vi "DAQ_pp3c_AllInit.vi"(8 "error in (no error)":errorcluster, 11 "Daq config in":T1={"Sound AO"="Dev6/ao0", "Shock intesity AO"="Dev6/ao1", "Code_LED DO"="Dev6/port1:2", "Switch DI"="Dev6/port0/line0", "Webcam"="cam9", "Sound AO task"="", "Sound card task"=0, "Shock intensity AO task"="", "Code_LED DO task"="", "Switch DI task"="", "AO <=> Sound card"=FALSE, "Sound card"=0, "sample rate"=100000.0, "Variable shock"=TRUE, "Webcam on"=FALSE, "Waveform memo"={"t0"=timestamp(0 s since 1904-01-01), "dt"=1.0, "Y"=[]}, "Tone trigger"="PFI1", "Master-9 DO"="PFI1", "Master-9 DO task"="Dev6/port0/line5:7", "Master-9 on"=TRUE} {"sample rate" min=8000.0; "Sound card task" format="%.0x"}) -> (0 "error out":errorcluster={"status"=FALSE, "code"=0, "source"="\n"}, 3 "Daq config out":T1={"Sound AO"="Dev6/ao0", "Shock intesity AO"="Dev6/ao1", "Code_LED DO"="Dev6/port1:2", "Switch DI"="Dev6/port0/line0", "Webcam"="cam9", "Sound AO task"="", "Sound card task"=0, "Shock intensity AO task"="", "Code_LED DO task"="", "Switch DI task"="", "AO <=> Sound card"=FALSE, "Sound card"=0, "sample rate"=100000.0, "Variable shock"=TRUE, "Webcam on"=FALSE, "Waveform memo"={"t0"=timestamp(0 s since 1904-01-01), "dt"=1.0, "Y"=[]}, "Tone trigger"="PFI1", "Master-9 DO"="PFI1", "Master-9 DO task"="Dev6/port0/line5:7", "Master-9 on"=TRUE} {"sample rate" min=8000.0; "Sound card task" format="%.0x"})   [LabVIEW 2013]
uses:
  CTL_pp3c_DaqStatus.ctl
  <vilib>/userdefined/High Color/IMAQdx.ctl
  <vilib>/sound2/lvsound2.llb/Sound Output Task ID.ctl
  <vilib>/sound2/lvsound2.llb/Sampling Mode.ctl
  <vilib>/sound2/lvsound2.llb/Sound Data Format.ctl
  <vilib>/DAQmx/write.llb/DAQmx Write (Digital U16 1Chan 1Samp).vi
  <vilib>/DAQmx/write.llb/DAQmx Write (Digital U32 1Chan 1Samp).vi
  <vilib>/DAQmx/create/channels.llb/DAQmx Create Channel (DO-Digital Output).vi
  <vilib>/DAQmx/create/channels.llb/DAQmx Create Channel (DI-Digital Input).vi
  <vilib>/DAQmx/create/channels.llb/DAQmx Create Channel (AO-Voltage-Basic).vi
  <vilib>/DAQmx/configure/timing.llb/DAQmx Timing (Sample Clock).vi
  <vilib>/DAQmx/miscellaneous.llb/DAQmx Fill In Error Info.vi
  <resource>/objmgr/daqmx.rc
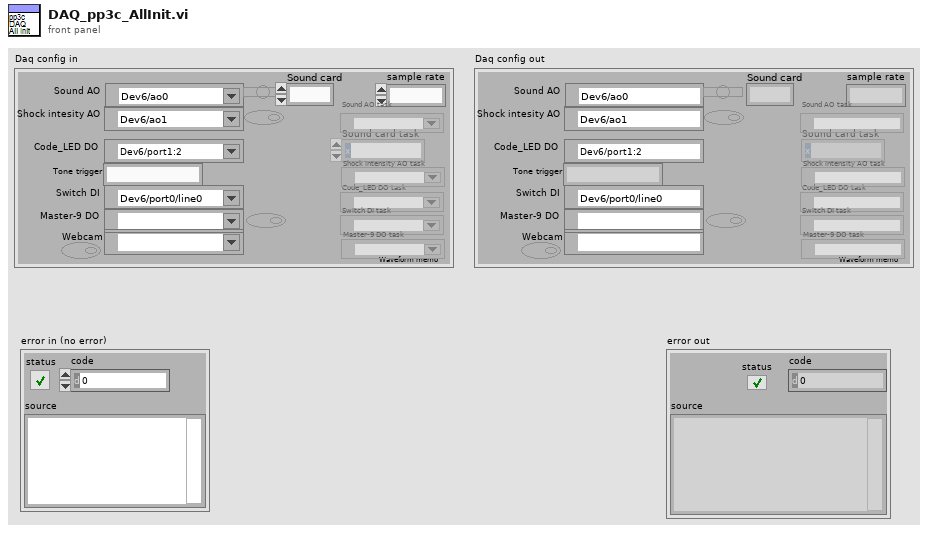
[diagram p1: front panel]
types:
  T1 = typedef "CTL_pp3c_DaqStatus.ctl" = cluster{"Sound AO":tag, "Shock intesity AO":tag, "Code_LED DO":tag, "Switch DI":tag, "Webcam":T2, "Sound AO task":refnum<k21>, "Sound card task":T3, "Shock intensity AO task":refnum<k21>, "Code_LED DO task":refnum<k21>, "Switch DI task":refnum<k21>, "AO <=> Sound card":bool, "Sound card":u32, "sample rate":dbl, "Variable shock":bool, "Webcam on":bool, "Waveform memo":waveform(dbl), "Tone trigger":string, "Master-9 DO":tag, "Master-9 DO task":refnum<k21>, "Master-9 on":bool}
  T2 = typedef "IMAQdx.ctl" = refnum<k21>
  T3 = typedef "Sound Output Task ID.ctl" = u32
  T4 = typedef "Sound Data Format.ctl" = cluster{"sample rate (S/s)":dbl, "number of channels":i32, "bits per sample":i32}
  T5 = typedef "Sampling Mode.ctl" = i32
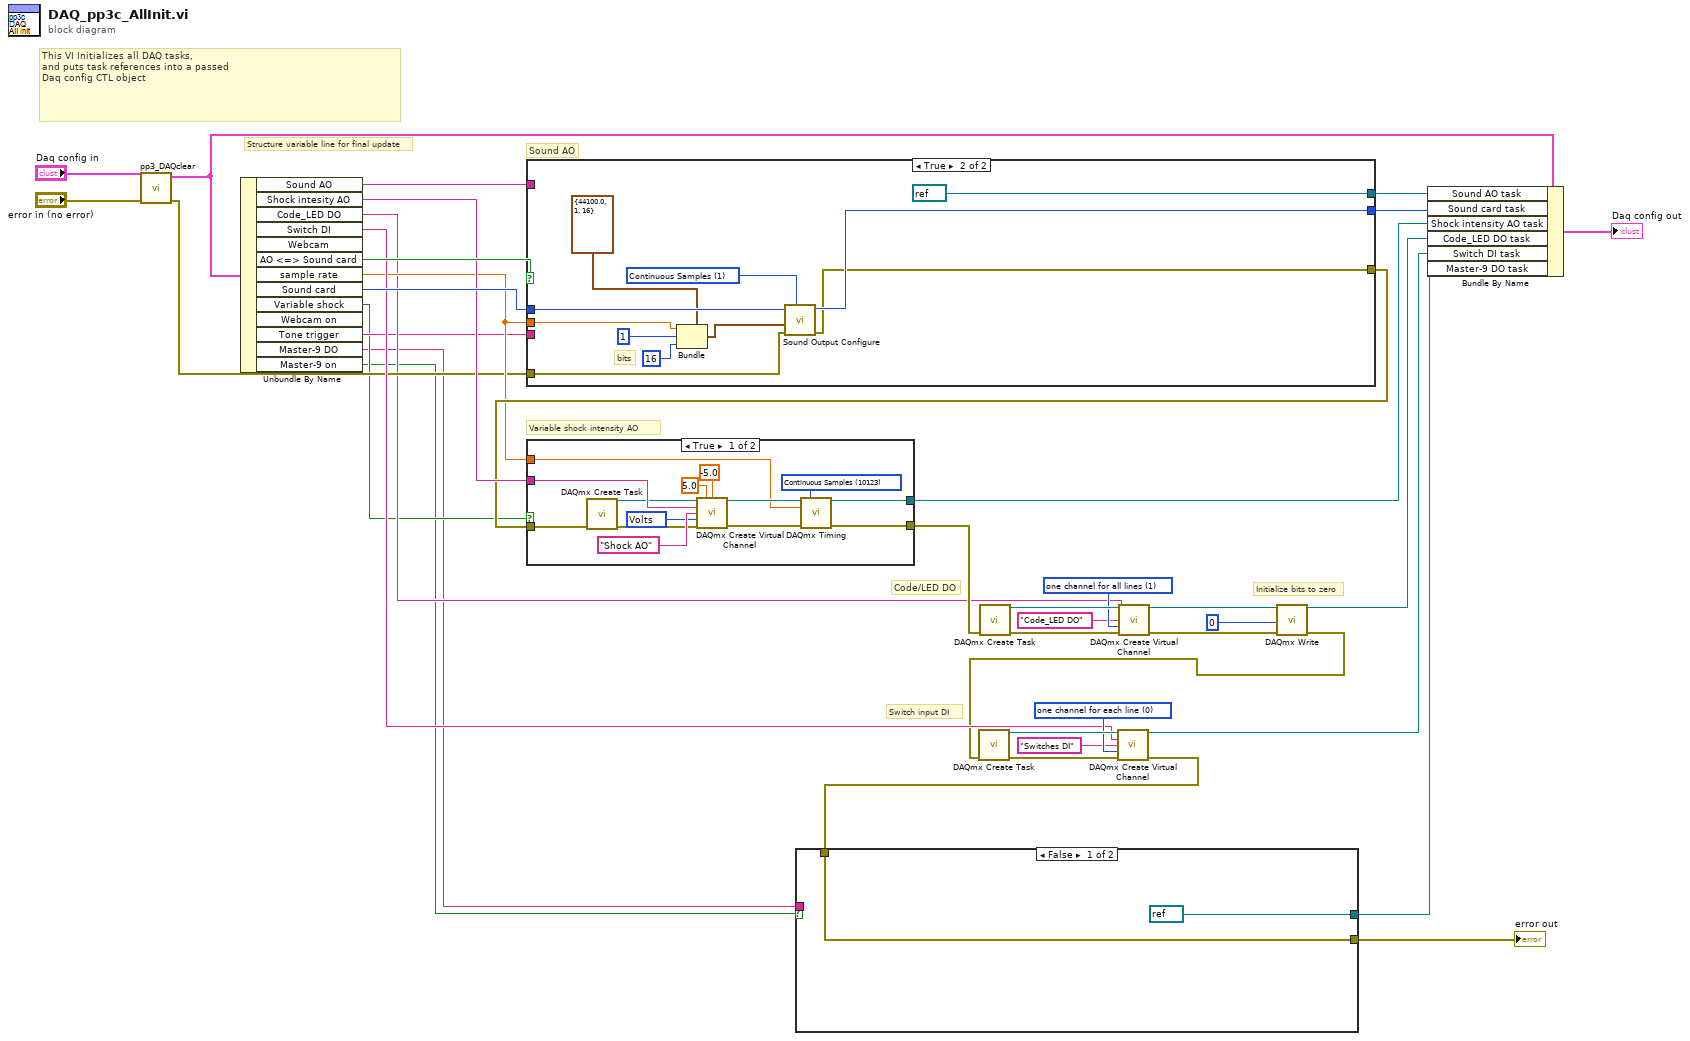
[diagram p0: block diagram]
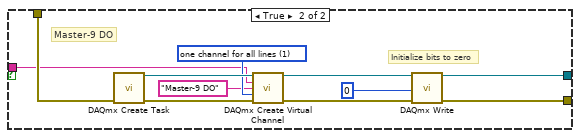
[diagram p2: hidden frame]
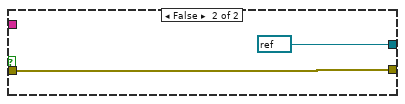
[diagram p3: hidden frame]
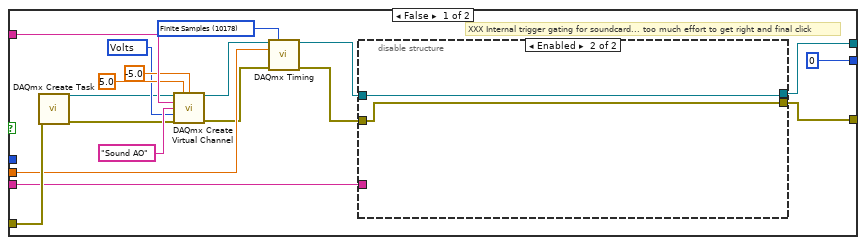
[diagram p4: hidden frame]
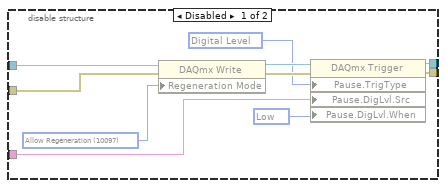
[diagram p5: hidden frame]
diagram:
  w24 = 0 items=["one channel for each line", "one channel for all lines"] ("line grouping")
  w28 = 1 items=["one channel for each line", "one channel for all lines"] ("line grouping")
  # "Initialize bits to zero"
  # "This VI Initializes all DAQ tasks,\nand puts task references into a passed\nDaq config CTL object"
  # "Switch input DI"
  # "Structure variable line for final update"
  # "Code/LED DO"
  # "Variable shock intensity AO"
  # "Sound AO"
  n1 = call "pp3_DAQclear.vi"("error in (no error)"="error in (no error)", "Daq config in"="Daq config in") -> ("error out"=w14:errorcluster, "Daq config out"=w16:T1)  [unwired: 8 in]
  n2 = Unbundle By Name(w16) -> ("Sound AO"=w37:tag, "Shock intesity AO"=w32:tag, "Code_LED DO"=w13:tag, "Switch DI"=w22:tag, "AO <=> Sound card"=w38:bool, "sample rate"=w18:dbl, "Sound card"=w34:u32, "Variable shock"=w11:bool, "Tone trigger"=w12:string, "Master-9 DO"=w2:tag, "Master-9 on"=w1:bool)  [unwired: 2 out]
  n3 = case shown="True" w38 {
    tunnel: w37 -> [w56 _]
    tunnel: [w46 refnum<k21> refnum ("task out")] -> w35
    tunnel: w34 -> [_ w78]
    tunnel: [T3 0 ("task ID") w74] -> w33
    tunnel: w14 -> [w50 w73]
    tunnel: [w45 w72] -> w20
    tunnel: w18 -> [w43 w71]
    tunnel: w12 -> [w47 _]
    frame False {
      w40 = 10178 items=["Finite Samples"=10178, "Continuous Samples"=10123, "Hardware Timed Single Point"=12522] ("sample mode")
      w51 = 10348 items=["Volts"=10348, "From Custom Scale"=10065] ("units")
      # "XXX Internal trigger gating for soundcard... too much effort to get right and final click"
      n4 = call <vilib>:"DAQmx Create Task.vi"("error in"=w50) -> ("task out"=w49:refnum<k21>, "error out"=w48:errorcluster)  [unwired: 13 in]
      n5 = call-poly <vilib>:"DAQmx Create Virtual Channel.vi"("task in"=w49, "maximum value"=5.0, "minimum value"=-5.0, "physical channels"=w56, "name to assign"="Sound AO", "units"=w51, "error in"=w48) -> ("task out"=w44:refnum<k21>, "error out"=w42:errorcluster)  [unwired: 7 in]
      n6 = call-poly <vilib>:"DAQmx Timing.vi"("task/channels in"=w44, "sample mode"=w40, "rate"=w43, "error in"=w42) -> ("task out"=w39:refnum<k21>, "error out"=w41:errorcluster)  [unwired: 10 in]
      n7 = disable-structure shown="Enabled" {
        disable-tunnel: w39 -> [w65 w68]
        disable-tunnel: w41 -> [w64 w67]
        disable-tunnel: w47 -> [w60 _]
        disable-tunnel: [w58 w68] -> w46
        disable-tunnel: [w57 w67] -> w45
        frame Disabled {
          w63 = 10214 items=["High"=10192, "Low"=10214] ("Pause.DigLvl.When")
          w59 = 10152 items=["Analog Level"=10101, "Analog Window"=10103, "Digital Level"=10152, "Digital Pattern"=10398, "None"=10230] ("Pause.TrigType")
          w66 = 10097 items=["Allow Regeneration"=10097, "Do Not Allow Regeneration"=10158] ("RegenMode")
          n8 = property class="DAQmx Write"(reference=w65, error in=w64, "Regeneration Mode"=w66) -> (reference out=w62:refnum<k21>, error out=w61:errorcluster)
          n9 = property class="DAQmx Trigger"(reference=w62, error in=w61, "Pause.TrigType"=w59, "Pause.DigLvl.Src"=w60, "Pause.DigLvl.When"=w63) -> (reference out=w58:refnum<k21>, error out=w57:errorcluster)
        }
        frame Enabled {
        }
      }
    }
    frame True {
      w77 = T5 1 items=["Finite Samples", "Continuous Samples"] ("sample mode")
      # "bits"
      n10 = Bundle(cluster=T4 {"sample rate (S/s)"=44100.0, "number of channels"=1, "bits per sample"=16} ("sound format"), "sample rate (S/s)"=w71, "number of channels"=1 ("Input.BufSize"), "bits per sample"=16 ("Input.BufSize")) -> (w69:T4)
      n11 = call <vilib>:"Sound Output Configure.vi"("sample mode"=w77, "error in (no error)"=w73, "sound format"=w69, "device ID"=w78) -> ("error out"=w72:errorcluster, "task ID"=w74:T3)  [unwired: 6 in]
    }
  }
  n12 = case shown="True" w11 {
    tunnel: w32 -> [w90 _]
    tunnel: [w84 refnum<k21> refnum ("task out")] -> w31
    tunnel: w18 -> [w86 _]
    tunnel: w20 -> [w82 w95]
    tunnel: [w83 w95] -> w19
    frame True {
      w85 = 10123 items=["Finite Samples"=10178, "Continuous Samples"=10123, "Hardware Timed Single Point"=12522] ("sample mode")
      w91 = 10348 items=["Volts"=10348, "From Custom Scale"=10065] ("units")
      n13 = call <vilib>:"DAQmx Create Task.vi"("error in"=w82) -> ("task out"=w80:refnum<k21>, "error out"=w81:errorcluster)  [unwired: 13 in]
      n14 = call-poly <vilib>:"DAQmx Create Virtual Channel.vi"("task in"=w80, "maximum value"=5.0, "minimum value"=-5.0, "physical channels"=w90, "name to assign"="Shock AO", "units"=w91, "error in"=w81) -> ("task out"=w88:refnum<k21>, "error out"=w87:errorcluster)  [unwired: 7 in]
      n15 = call-poly <vilib>:"DAQmx Timing.vi"("task/channels in"=w88, "sample mode"=w85, "rate"=w86, "error in"=w87) -> ("task out"=w84:refnum<k21>, "error out"=w83:errorcluster)  [unwired: 10 in]
    }
    frame False {
    }
  }
  n16 = call <vilib>:"DAQmx Create Task.vi"("error in"=w19) -> ("task out"=w29:refnum<k21>, "error out"=w30:errorcluster)  [unwired: 13 in]
  n17 = call-poly <vilib>:"DAQmx Create Virtual Channel.vi"("task in"=w29, "lines"=w13, "name to assign"="Code_LED DO", "line grouping"=w28, "error in"=w30) -> ("task out"=w9:refnum<k21>, "error out"=w7:errorcluster)  [unwired: 9 in]
  n18 = call-poly <vilib>:"DAQmx Write.vi"("task/channels in"=w9, "data"=u16 0, "error in"=w7) -> ("task out"=w8:refnum<k21>, "error out"=w5:errorcluster)  [unwired: 10 in, 1 out]
  n19 = call <vilib>:"DAQmx Create Task.vi"("error in"=w5) -> ("task out"=w25:refnum<k21>, "error out"=w26:errorcluster)  [unwired: 13 in]
  n20 = call-poly <vilib>:"DAQmx Create Virtual Channel.vi"("task in"=w25, "lines"=w22, "name to assign"="Switches DI", "line grouping"=w24, "error in"=w26) -> ("task out"=w21:refnum<k21>, "error out"=w10:errorcluster)  [unwired: 9 in]
  n21 = case shown="False" w1 {
    tunnel: w10 -> [w96 w104]
    tunnel: [w96 w102] -> w4
    tunnel: [refnum<k21> refnum ("task out") w101] -> w3
    tunnel: w2 -> [_ w98]
    frame False {
    }
    frame True {
      w106 = 1 items=["one channel for each line", "one channel for all lines"] ("line grouping")
      # "Initialize bits to zero"
      # "Master-9 DO"
      n22 = call <vilib>:"DAQmx Create Task.vi"("error in"=w104) -> ("task out"=w107:refnum<k21>, "error out"=w108:errorcluster)  [unwired: 13 in]
      n23 = call-poly <vilib>:"DAQmx Create Virtual Channel.vi"("task in"=w107, "lines"=w98, "name to assign"="Master-9 DO", "line grouping"=w106, "error in"=w108) -> ("task out"=w100:refnum<k21>, "error out"=w99:errorcluster)  [unwired: 9 in]
      n24 = call-poly <vilib>:"DAQmx Write.vi"("task/channels in"=w100, "data"=u32 0, "error in"=w99) -> ("task out"=w101:refnum<k21>, "error out"=w102:errorcluster)  [unwired: 10 in, 1 out]
    }
  }
  "error out" <- w4
  n25 = Bundle By Name(cluster=w16, "Sound AO task"=w35, "Sound card task"=w33, "Shock intensity AO task"=w31, "Code_LED DO task"=w8, "Switch DI task"=w21, "Master-9 DO task"=w3) -> (→"Daq config out":T1)
